vi "Visualization_Init.vi"() -> (0 "error out":errorcluster, 3 "visualization out":refnum<class "Visualization.lvclass">)   [LabVIEW 2018]
uses:
  <vilib>/Quanser/Rapid Control Prototyping Toolkit/visualization/Visualization.lvclass
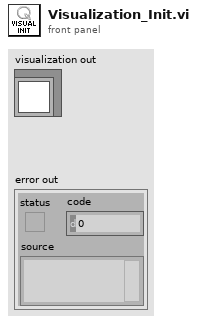
[diagram p1: front panel]
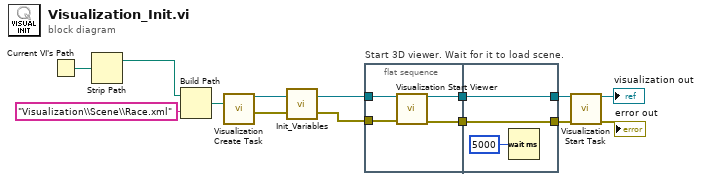
[diagram p0: block diagram]
diagram:
  n1 = Current VI's Path() -> (path=w9:path)
  n2 = Strip Path(path=w9) -> (stripped path=w1:path)  [unwired: 1 out]
  n3 = Build Path(base path=w1, name or relative path="Visualization\\Scene\\Race.xml") -> (appended path=w11:path)
  n4 = call <vilib>:"Visualization Create Task.vi"("scene filename"=w11) -> ("visualization out"=w5:refnum<class "Visualization.lvclass">, "error out"=w4:errorcluster)  [unwired: 13 in]
  n5 = call "Init_Variables.vi"("error in"=w4, "task in"=w5) -> ("error out"=w2:errorcluster, "task out"=w3:refnum<class "Visualization.lvclass">)
  n6 = flat-sequence "Start 3D viewer. Wait for it to load scene." {
    tunnel: w3 -> [w16]
    tunnel: w2 -> [w17]
    tunnel: [w18] -> w14
    tunnel: [w15] -> w13
    tunnel: [w21] -> w8
    tunnel: [w19] -> w12
    tunnel: w14 -> [w21]
    tunnel: w13 -> [w19]
    frame #0 {
      n7 = call <vilib>:"Visualization Start Viewer.vi"("visualization in"=w16, "error in (no error)"=w17) -> ("visualization out"=w15:refnum<class "Visualization.lvclass">, "error out"=w18:errorcluster)  [unwired: 12 in]
    }
    frame #1 {
      n8 = Wait (ms)(milliseconds to wait=u32 5000) -> ()  [unwired: 1 out]
    }
  }
  n9 = call <vilib>:"Visualization Start Task.vi"("visualization in"=w12, "error in (no error)"=w8) -> ("visualization out"=→"visualization out":refnum<class "Visualization.lvclass">, "error out"=→"error out":errorcluster)  [unwired: 12 in]
